vi "Optomize Settings.vi"(5 "Aviod Zone":cluster{"pos 1":dbl, "pos 2":dbl} {"pos 1" format="%#.3g"; "pos 2" format="%#.3g"}, 7 "Previous Swerve Setting":T1 {"Back Right"."Angle" scale format="%.3f"; "Back Right"."Velocity" scale=-1.0..1.0 scale format="%.1f"; "Back Left"."Angle" scale format="%.3f"; "Back Left"."Velocity" scale=-1.0..1.0 scale format="%.1f"; "Front Left"."Angle" scale format="%.3f"; "Front Left"."Velocity" scale=-1.0..1.0 scale format="%.1f"; "Front Right"."Angle" scale format="%.3f"; "Front Right"."Velocity" scale=-1.0..1.0 scale format="%.1f"}, 11 "Swerve Request":T1 {"Back Right"."Angle" scale format="%.3f"; "Back Right"."Velocity" scale=-1.0..1.0 scale format="%.1f"; "Back Left"."Angle" scale format="%.3f"; "Back Left"."Velocity" scale=-1.0..1.0 scale format="%.1f"; "Front Left"."Angle" scale format="%.3f"; "Front Left"."Velocity" scale=-1.0..1.0 scale format="%.1f"; "Front Right"."Angle" scale format="%.3f"; "Front Right"."Velocity" scale=-1.0..1.0 scale format="%.1f"}) -> (3 "Swerve Setting Out":T1 {"Back Right"."Angle" scale format="%.3f"; "Back Right"."Velocity" scale=-1.0..1.0 scale format="%.1f"; "Back Left"."Angle" scale format="%.3f"; "Back Left"."Velocity" scale=-1.0..1.0 scale format="%.1f"; "Front Left"."Angle" scale format="%.3f"; "Front Left"."Velocity" scale=-1.0..1.0 scale format="%.1f"; "Front Right"."Angle" scale format="%.3f"; "Front Right"."Velocity" scale=-1.0..1.0 scale format="%.1f"})   [LabVIEW 2023, in "SwerveDrive_ACT_ts.lvlib"]
uses:
  SwerveDrive_ACT_ts.lvlib
  Shared Code/TypeDefs/Cluster_Swerve 4 Steer and Velocity.ctl
  Shared Code/TypeDefs/Cluster_Module Velocity-Direction-Rotations.ctl
  Shared Code/TypeDefs/Level_Velocity plus-minus 1.ctl
  Shared Code/TypeDefs/Dial_Compase heading unit circle CCW positive.ctl
panel:
  # "\"Front\" of Robot"
  # "Right Hand Rule"
  # "X"
  # "+CCW"
  # "Y"
  # "(0,0)"
  # "\"Front\" of Robot"
  # "Right Hand Rule"
  # "X"
  # "+CCW"
  # "Y"
  # "(0,0)"
  # "\"Front\" of Robot"
  # "Right Hand Rule"
  # "X"
  # "+CCW"
  # "Y"
  # "(0,0)"
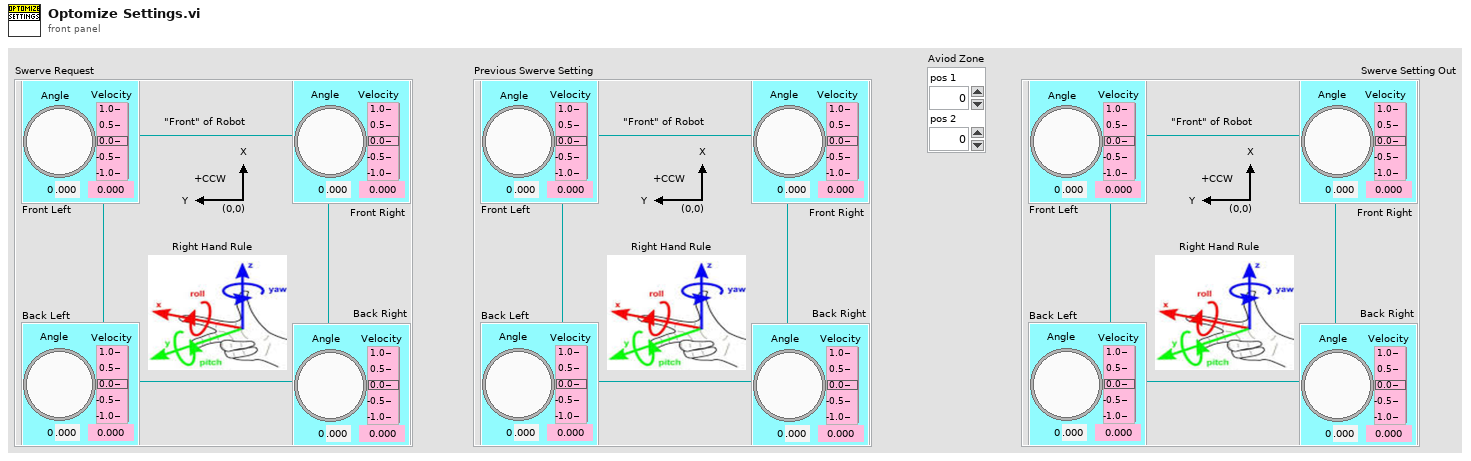
[diagram p1: front panel]
types:
  T1 = typedef "Cluster_Swerve 4 Steer and Velocity.ctl" = cluster{"Front Right":T2, "Front Left":T2, "Back Left":T2, "Back Right":T2}
  T2 = typedef "Cluster_Module Velocity-Direction-Rotations.ctl" = cluster{"Velocity":T3, "Angle":T4, "Rotations Count":dbl}
  T3 = typedef "Level_Velocity plus-minus 1.ctl" = dbl
  T4 = typedef "Dial_Compase heading unit circle CCW positive.ctl" = dbl
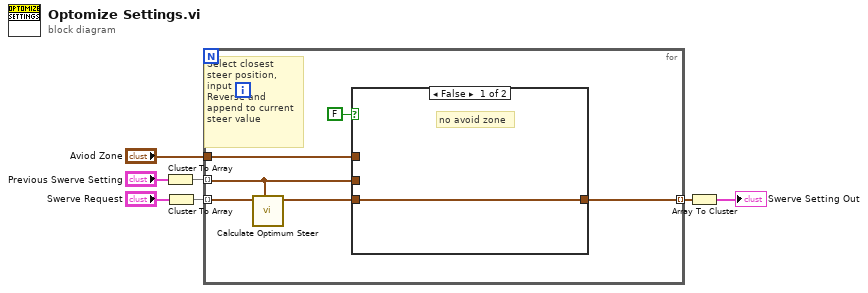
[diagram p0: block diagram]
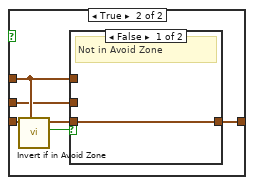
[diagram p2: hidden frame]
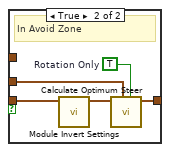
[diagram p3: hidden frame]
diagram:
  n1 = Cluster To Array(cluster="Previous Swerve Setting") -> (array=w3:T2[])
  n2 = Cluster To Array(cluster="Swerve Request") -> (array=w5:T2[])
  n3 = for {
    tunnel: w5 -> [w9] mode=indexing
    tunnel: "Aviod Zone" -> [w12]
    tunnel: w3 -> [w11] mode=indexing
    tunnel: [w10] -> w2 mode=indexing
    # "Select closest\nsteer position,\ninput or\nReverse and\nappend to current\nsteer value"
    n4 = call "Calculate Optimum Steer.vi"("Previous Set Swerve"=w11, "New Swerve"=w9) -> ("Set Swerve Out"=w13:T2)  [unwired: 9 in]
    n5 = case shown="False" FALSE {
      tunnel: w13 -> [w14 w20]
      tunnel: w12 -> [_ w18]
      tunnel: w11 -> [_ w17]
      tunnel: [w14 w16] -> w10
      frame False {
        # "no avoid zone"
      }
      frame True {
        n6 = call "Invert if in Avoid Zone.vi"("Avoid Zone (Unit Circle)"=w18, "Set Values"=w20) -> ("In Avoid Zone"=w19:bool, "Set Values Out"=w15:T2)  [unwired: 8 in]
        n7 = case shown="False" w19 {
          tunnel: w18 -> [_ _]
          tunnel: w17 -> [_ w26]
          tunnel: [w21 w25] -> w16
          tunnel: w15 -> [w21 w23]
          frame False {
            # "Not in Avoid Zone"
          }
          frame True {
            w22 = TRUE  # Rotation Only
            # "In Avoid Zone"
            n8 = call "Module Invert Settings.vi"("Setting"=w23) -> ("Inverted Setting Out"=w24:T2)  [unwired: 10 in]
            n9 = call "Calculate Optimum Steer.vi"("Rotation Only"=w22, "Previous Set Swerve"=w26, "New Swerve"=w24) -> ("Set Swerve Out"=w25:T2)  [unwired: 8 in]
          }
        }
      }
    }
  }
  n10 = Array To Cluster(array=w2) -> (cluster=→"Swerve Setting Out":cluster{"[0]":T2, "[1]":T2, "[2]":T2, "[3]":T2})
